vi "Left Click.vi"(7 "object refs":T2, 8 "error in":errorcluster, 9 "Coords":T1, 10 "Event data":variant, 11 "Multi Column Listbox in":refnum<class "Multi Column Listbox.lvclass">) -> (0 "error out":errorcluster, 2 "Discard?":bool, 3 "Multi Column Listbox out":refnum<class "Multi Column Listbox.lvclass">)   [LabVIEW 2014, in "Table Manager.lvlib" / "Multi Column Listbox.lvclass"]
uses:
  Multi Column Listbox.lvclass
  Table Manager/object ref.ctl
  Configuration Editor/Classes/Engine Parent/Engine Parent Editor Node.lvclass
  Configuration Editor/Classes/Module editor node/module editor node.lvclass
  <vilib>/Utility/miscctls.llb/LVPoint32TypeDef.ctl
  Multi Column Listbox.lvclass/Multi Column Listbox.ctl
  Table Manager/Table Manager.lvclass/Table Manager.ctl
  Line/Line.lvclass/Line.ctl
  Column/Column.lvclass/Column.ctl
  Line/Read Columns.vi
  Line/Write Columns.vi
  Read Listbox.vi
  Table Manager/Read Line.vi
  Table Manager/Read Top VI.vi
  Table Manager/Write Line.vi
  Line/Line.lvclass
  Column/Column.lvclass
  Table Manager/Table Manager.lvclass
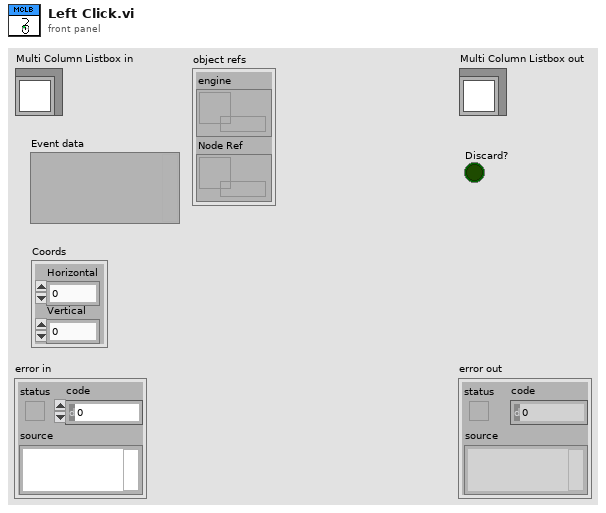
[diagram p1: front panel]
types:
  T1 = typedef "LVPoint32TypeDef.ctl" = cluster{"Horizontal":i32, "Vertical":i32}
  T2 = typedef "Table Manager.lvlib/Table Manager.lvclass/object ref.ctl" = cluster{"engine":refnum<data-value>, "Node Ref":refnum<data-value>}
  T3 = typedef "LVRowAndColumnTypeDef.ctl" = cluster{"Row":i32, "Column":i32}
  T4 = typedef "LVPositionTypeDef.ctl" = cluster{"Left":i32, "Top":i32}
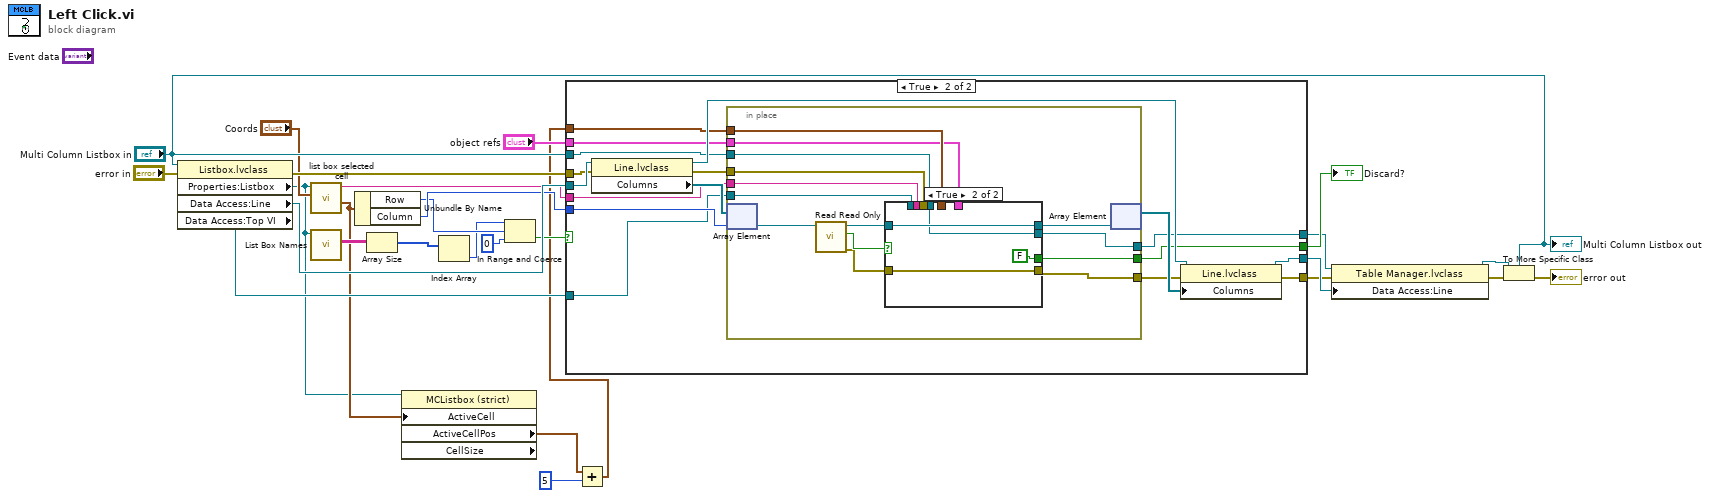
[diagram p0: block diagram]
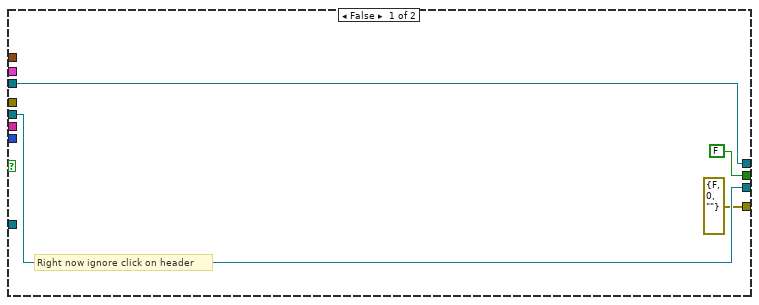
[diagram p2: hidden frame]
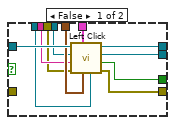
[diagram p3: hidden frame]
diagram:
  n1 = property class="Listbox.lvclass"(reference="Multi Column Listbox in", error in="error in") -> (error out=w9:errorcluster, "Properties:Listbox"=w4:refnum<vi>, "Data Access:Line"=w27:refnum<class "Line.lvclass">, "Data Access:Top VI"=w7:refnum<vi>)  [unwired: 1 out]
  n2 = call "list box selected cell.vi"("Coords"="Coords", "MulticolumnListbox in"=w4) -> ("cell position"=w5:T3, "tag select name"=w16:string)  [unwired: 6 in, 2 out]
  n3 = call "List Box Names.vi"("MulticolumnListbox in"=w4) -> ("ItemNames"=w22:string[][])  [unwired: 8 in, 2 out]
  n4 = Unbundle By Name(w5) -> ("Row"=w24:i32, "Column"=w26:i32)
  n5 = Array Size(array=w22) -> (size(s)=w21:i32[])
  n6 = property class="MCListbox (strict)" props=["ActiveCell", "ActiveCellPos", "CellSize"](reference=w4, "ActiveCell"=w5) -> ("ActiveCellPos"=w3:T4)  [unwired: 1 in, 3 out]
  n7 = Index Array(array=w21) -> (element=w20:i32)  [unwired: 1 in]
  n8 = In Range and Coerce(upper limit=w20, x=w24, lower limit=0) -> (In Range?=w25:bool)  [unwired: 1 out]
  n9 = Add(x=w3, y=5) -> (x+y=w1:T4)
  n10 = case shown="True" w25 {
    tunnel: w27 -> [w31 w48]
    tunnel: w26 -> [_ w47]
    tunnel: [w31 w43] -> w19
    tunnel: [errorcluster {"status"=FALSE, "code"=0, "source"=""} ("error out") w42] -> w18
    tunnel: [FALSE ("Discard") w41] -> w17
    tunnel: w1 -> [_ w40]
    tunnel: w16 -> [_ w39]
    tunnel: "Multi Column Listbox in" -> [w28 w38]
    tunnel: [w28 w37] -> w15
    tunnel: "object refs" -> [_ w36]
    tunnel: w9 -> [_ w33]
    tunnel: w7 -> [_ w32]
    frame False {
      # "Right now ignore click on header"
    }
    frame True {
      n11 = property class="Line.lvclass"(reference=w48, error in=w33) -> (reference out=w44:refnum<class "Line.lvclass">, error out=w35:errorcluster, "Columns"=w46:refnum<class "Column.lvclass">[])
      n12 = in-place {
        in-place-border: [w61] -> w41
        in-place-border: w40 -> [w60]
        in-place-border: w32 -> [w59]
        in-place-border: w39 -> [w58]
        in-place-border: w38 -> [w57]
        in-place-border: [w56] -> w37
        in-place-border: w36 -> [w55]
        in-place-border: w35 -> [w54]
        in-place-border: [w53] -> w34
        n13 = in-place-array #1(w46, w47) -> (w52:refnum<class "Column.lvclass">)
        n14 = call "Read Read Only.vi"("Column in"=w52) -> ("error out"=w49:errorcluster, "Read Only"=w50:bool, "Column out"=w51:refnum<class "Column.lvclass">)  [unwired: 8 in]
        n15 = case shown="True" w50 {
          tunnel: w51 -> [w73 w76]
          tunnel: [w72 w76] -> w62
          tunnel: [w71 FALSE ("Discard")] -> w61
          tunnel: w60 -> [w70 _]
          tunnel: w59 -> [w69 _]
          tunnel: w58 -> [w68 _]
          tunnel: w57 -> [w67 w75]
          tunnel: [w66 w75] -> w56
          tunnel: w55 -> [w65 _]
          tunnel: w54 -> [w64 _]
          tunnel: [w63 w74] -> w53
          tunnel: w49 -> [_ w74]
          frame False {
            n16 = call-dynamic "Left Click.vi"("Top  VI"=w69, "Coords"=w70, "object refs"=w65, "error in (no error)"=w64, "line name"=w68, "Table Manager in"=w67, "column in"=w73) -> ("error out"=w63:errorcluster, "Discard"=w71:bool, "Table Manager out"=w66:refnum<class "Table Manager.lvclass">, "column out"=w72:refnum<class "Column.lvclass">)  [unwired: 1 in]
          }
          frame True {
          }
        }
        n17 = in-place-array #1(w62) -> (w45:refnum<class "Column.lvclass">[])  [unwired: 1 out]
      }
      n18 = property class="Line.lvclass"(reference=w44, error in=w34, "Columns"=w45) -> (reference out=w43:refnum<class "Line.lvclass">, error out=w42:errorcluster)
    }
  }
  "Discard?" <- w17
  n19 = property class="Table Manager.lvclass"(reference=w15, error in=w18, "Data Access:Line"=w19) -> (reference out=w13:refnum<class "Table Manager.lvclass">, error out=w12:errorcluster)
  n20 = To More Specific Class(target class="Multi Column Listbox in", reference=w13, error in=w12) -> (error out=→"error out":errorcluster)  [unwired: 1 out]
  "Multi Column Listbox out" <- "Multi Column Listbox in"
